vi "control_visualizations.vi"() -> ()   [LabVIEW 2019]
panel:
  out "OK Button":bool
  out "OK Button 5":bool
  out "OK Button 4":bool
  in  "Boolean":bool
  out "OK Button 3":bool
  out "OK Button 2":bool
  out "Slide 2":dbl(slide) scale=0.0..100.0
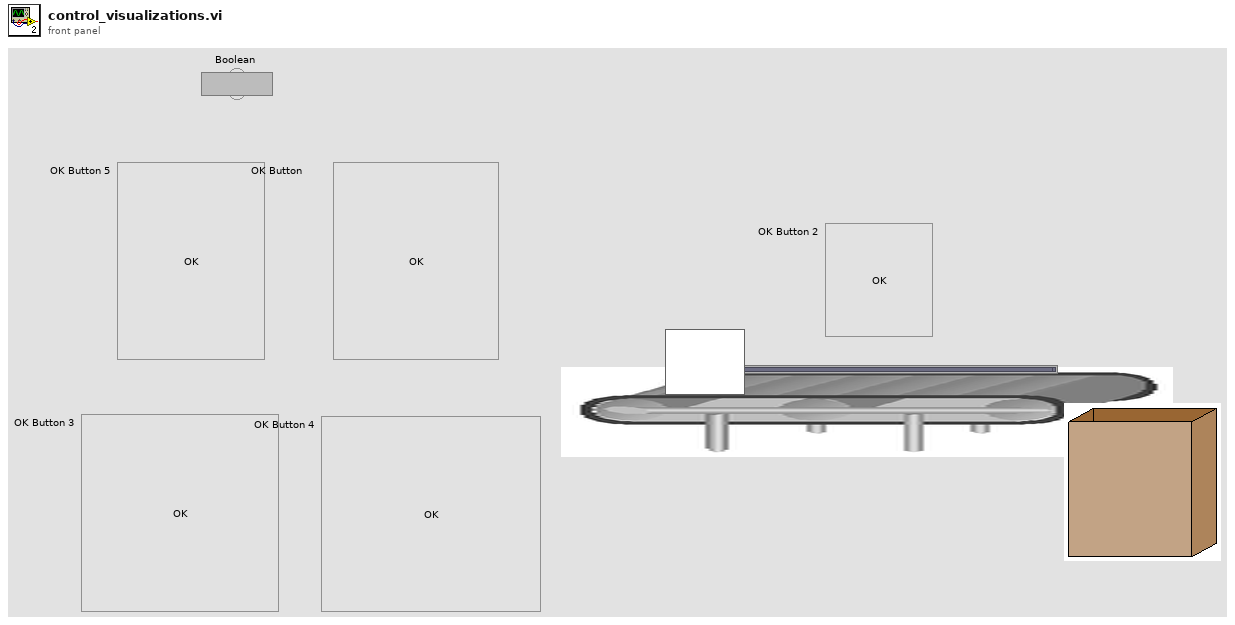
[diagram p1: front panel]
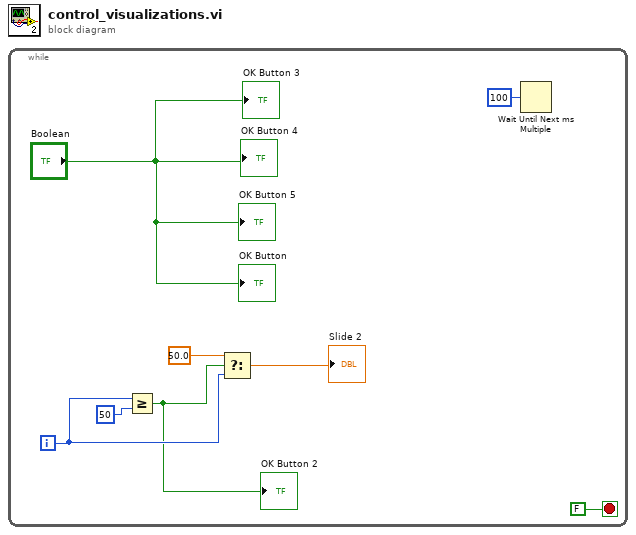
[diagram p0: block diagram]
diagram:
  n1 = while {
    i -> [w4]
    stop <- FALSE stop-if-true
    n2 = Greater Or Equal?(x=w4, y=50) -> (x >= y?=w2:bool)
    "OK Button 2" <- w2
    n3 = Select(t=50.0, s=w2, f=w4) -> (s? t:f=→"Slide 2":dbl)
    n4 = Wait Until Next ms Multiple(millisecond multiple=u32 100) -> ()  [unwired: 1 out]
    "OK Button 3" <- "Boolean"
    "OK Button 4" <- "Boolean"
    "OK Button 5" <- "Boolean"
    "OK Button" <- "Boolean"
  }
